vi "Build OPCUA Variable Name.vi"(10 "Varible Sub Name":string, 11 "Varible Header Name":string) -> (3 "resulting string":string)   [LabVIEW 2021]
panel:
  out "unsigned byte array":u8[](array[numeric])
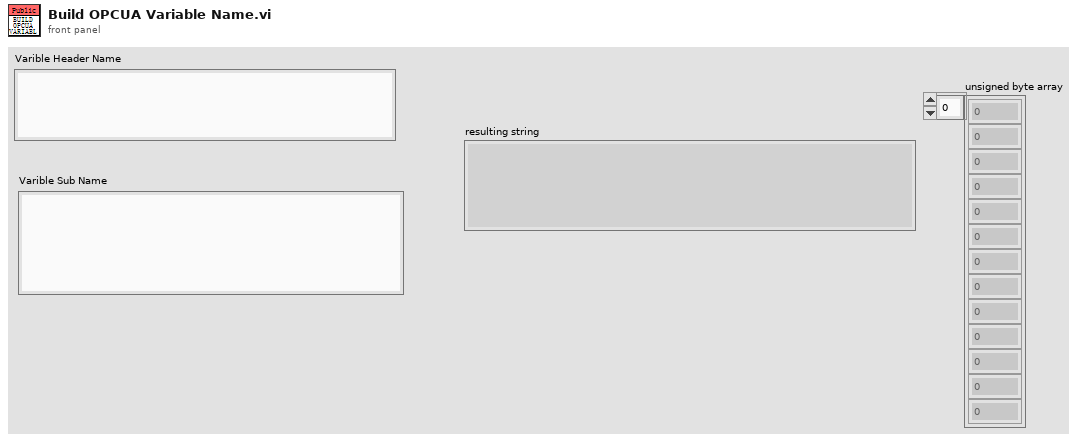
[diagram p1: front panel]
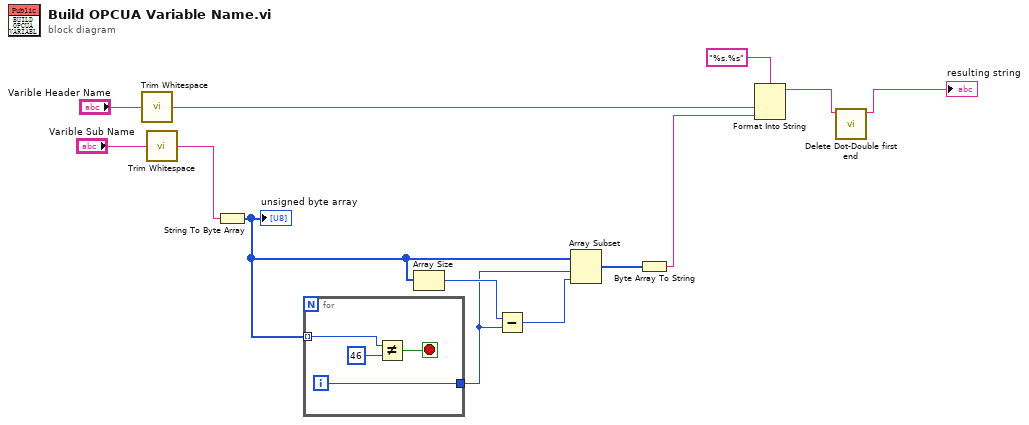
[diagram p0: block diagram]
diagram:
  n1 = call <vilib>:"Trim Whitespace.vi"("string"="Varible Header Name") -> ("trimmed string"=w10:string)  [unwired: 1 in]
  n2 = call <vilib>:"Trim Whitespace.vi"("string"="Varible Sub Name") -> ("trimmed string"=w4:string)  [unwired: 1 in]
  n3 = String To Byte Array(string=w4) -> (unsigned byte array=w9:u8[])
  "unsigned byte array" <- w9
  n4 = for {
    tunnel: w9 -> [w17] mode=indexing
    tunnel: [w14] -> w7
    i -> [w14]
    stop <- w15 stop-if-true
    n5 = Not Equal?(x=w17, y=u8 46) -> (x != y?=w15:bool)
  }
  n6 = Array Size(array=w9) -> (size(s)=w8:i32)
  n7 = Subtract(x=w8, y=w7) -> (x-y=w6:i32)
  n8 = Array Subset(array=w9, index=w7, length=w6) -> (w5:u8[])
  n9 = Byte Array To String(unsigned byte array=w5) -> (string=w3:string)
  n10 = Format Into String(format string="%s.%s", w10, w3) -> (resulting string=w2:string)  [unwired: 2 in, 1 out]
  n11 = call "Delete Dot-Double first end.vi"("String"=w2) -> ("string"=→"resulting string":string)  [unwired: 10 in]
